vi "estimador velocidade robo.vi"(11 "Detection Robot":T1 {"height" format="%+4.3f"; "pixel_y" format="%+4.3f"; "pixel_x" format="%+4.3f"; "orientation" format="%+4.3f"; "y" format="%+4.3f"; "confidence" format="%4.3f"; "x" format="%+4.3f"}) -> (1 "angular speed (rad/s)":dbl, 2 "v_y (cm/s)":dbl, 3 "v_x (cm/s)":dbl)   [LabVIEW 2016]
uses:
  SSL Detection Robot.ctl
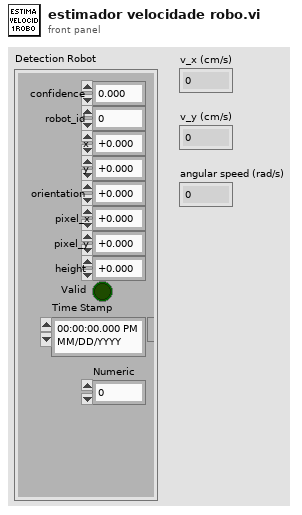
[diagram p1: front panel]
types:
  T1 = typedef "SSL Detection Robot.ctl" = cluster{"x":dbl, "robot_id":u32, "confidence":sgl, "y":sgl, "orientation":sgl, "pixel_x":sgl, "pixel_y":sgl, "height":sgl, "Valid":bool, "Time Stamp":timestamp, "Numeric":dbl}
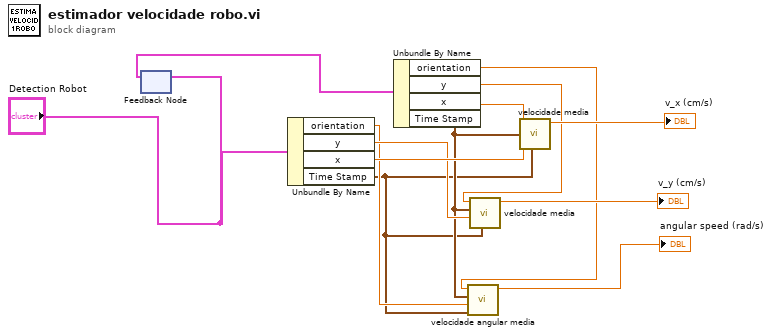
[diagram p0: block diagram]
diagram:
  n1 = feedback #1() -> (w13:T1)  [unwired: 1 in]
  n2 = feedback-in #1("Detection Robot") -> ()
  n3 = Unbundle By Name("Detection Robot") -> ("orientation"=w5:sgl, "y"=w8:sgl, "x"=w11:dbl, "Time Stamp"=w3:timestamp)
  n4 = Unbundle By Name(w13) -> ("orientation"=w6:sgl, "y"=w9:sgl, "x"=w12:dbl, "Time Stamp"=w4:timestamp)
  n5 = call "velocidade angular media.vi"("Time Stamp 2"=w3, "tetha 2"=w5, "Time Stamp 1"=w4, "tetha 1"=w6) -> ("angular speed (rad/s)"=→"angular speed (rad/s)":dbl)  [unwired: 7 in]
  n6 = call "velocidade media.vi"("Time Stamp 2"=w3, "x 2"=w8, "Time Stamp 1"=w4, "x1"=w9) -> ("speed (cm/s)"=→"v_y (cm/s)":dbl)  [unwired: 7 in]
  n7 = call "velocidade media.vi"("Time Stamp 2"=w3, "x 2"=w11, "Time Stamp 1"=w4, "x1"=w12) -> ("speed (cm/s)"=→"v_x (cm/s)":dbl)  [unwired: 7 in]
